vi "Feedback Node - Setting a Delay Value.vi"() -> ()   [LabVIEW 2023]
doc: "Demonstrates the use of a \"Delay\" value on a Feedback Node to store multiple iterations worth of data. This is analogous to showing multiple elements on a shift register."
panel:
  out "Multiple Delay Output (Shift Register)":i32[](graph)
  out "Multiple Delay Output (Feedback Node)":i32[](graph)
  # "Overview: Demonstrates the configuration of a Delay value on a Feedback Node to store multiple iterations worth of data.\nInstructions:\nRun the VI. It shows that a feedback node with a delay functions identically to a shift register with multiple elements. See the block diagram for more information."
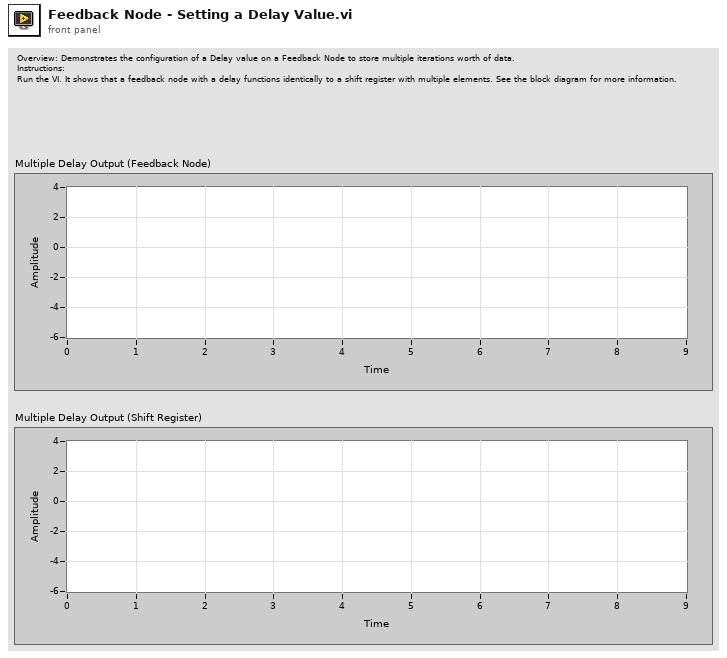
[diagram p1: front panel]
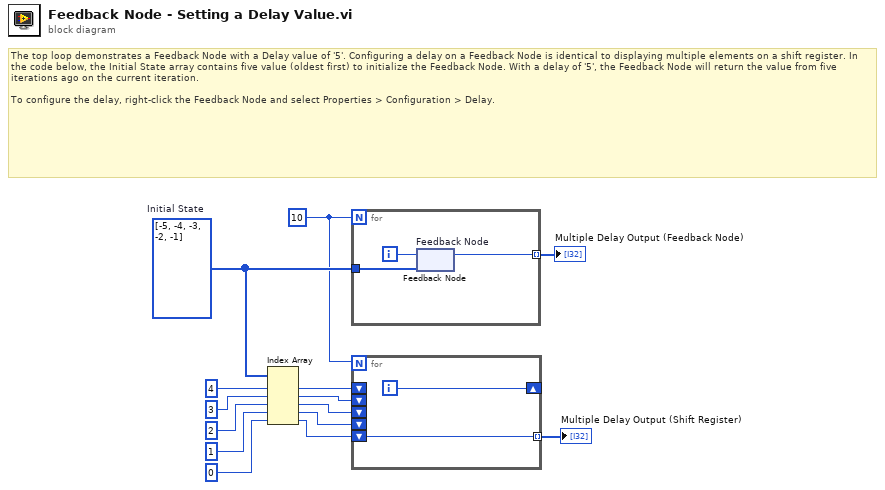
[diagram p0: block diagram]
diagram:
  w12 = i32[] [-5, -4, -3, -2, -1]  # Initial State
  w6 = 10
  # "The top loop demonstrates a Feedback Node with a Delay value of '5'. Configuring a delay on a Feedback Node is identical to displaying multiple elements on a shift register. In the code below, the Initial State array contains five value (oldest first) to initialize the Feedback Node. With a delay of '5', the Feedback Node will return the value from five iterations ago on the current iteration.\n\nTo configure the delay, right-click the Feedback Node and select Properties > Configuration > Delay."
  n1 = Index Array(array=w12, index #1=4 ("index"), index #2=3 ("index"), index #3=2 ("index"), index #4=1 ("index"), index #5=0 ("index")) -> (element #1=w11:i32, element #2=w10:i32, element #3=w9:i32, element #4=w8:i32, element #5=w7:i32)
  n2 = for {
    N: w6 -> [_]
    tunnel: [w16] -> w14 mode=indexing
    tunnel: w12 -> [w17]
    i -> [w15]
    n3 = feedback-in #1(w15) -> ()
    n4 = feedback #1 "Feedback Node"(w17) -> (w16:i32)
  }
  "Multiple Delay Output (Feedback Node)" <- w14
  n5 = for {
    N: w6 -> [_]
    tunnel: [w19] -> w13 mode=indexing
    shift-right: [w18] -> _
    shift-left: w11 -> [_]
    shift-left: w10 -> [_]
    shift-left: w9 -> [_]
    shift-left: w8 -> [_]
    shift-left: w7 -> [w19]
    i -> [w18]
  }
  "Multiple Delay Output (Shift Register)" <- w13
